vi "Extract strain.vi"() -> ()   [LabVIEW 2015]
uses:
  <vilib>/Utility/file.llb/Read From Spreadsheet File (DBL).vi
panel:
  in  "File Path Control":path
  out "Waveform Graph":dbl[][](graph)
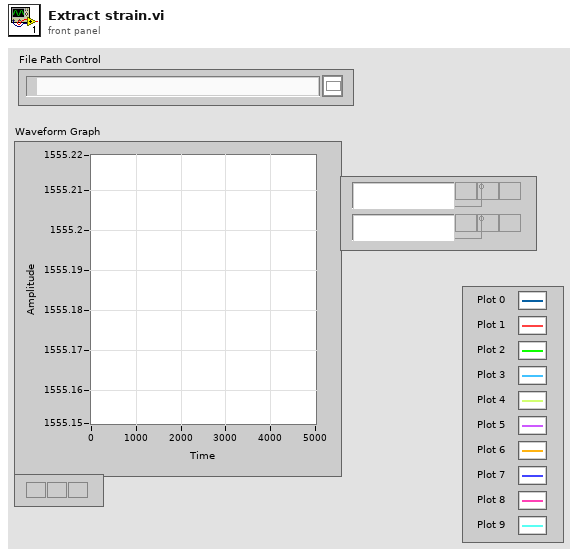
[diagram p1: front panel]
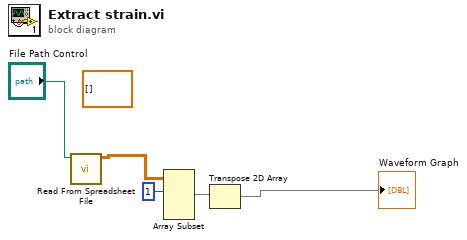
[diagram p0: block diagram]
diagram:
  (unwired) dbl[][] []
  n1 = call-poly <vilib>:"Read From Spreadsheet File.vi"("file path (dialog if empty)"="File Path Control") -> ("all rows"=w4:dbl[][])  [unwired: 6 in, 4 out]
  n2 = Array Subset(array=w4, index (row)=1 ("index")) -> (w3:dbl[][])  [unwired: 3 in]
  n3 = Transpose 2D Array(2D array=w3) -> (transposed array=→"Waveform Graph":dbl[][])
